vi "MasterAcquisitionFile_IOS_GCaMP_Garborg.vi"() -> ()   [LabVIEW 2020]
uses:
  <vilib>/vision/driver/IMAQdx.llb/IMAQdx Camera Control Mode.ctl
  <vilib>/vision/driver/IMAQdx.llb/IMAQdx Acquisition Mode.ctl
  <vilib>/userDefined/High Color/IMAQdx.ctl
  <vilib>/vision/driver/IMAQdx.llb/IMAQdx Buffer Number Mode.ctl
  <vilib>/DAQmx/write.llb/DAQmx Write (Digital 1D Wfm NChan NSamp).vi
  <vilib>/DAQmx/write.llb/DAQmx Write (Digital Bool 1Line 1Point).vi
  <vilib>/DAQmx/read.llb/DAQmx Read (Analog 1D Wfm NChan NSamp).vi
  <vilib>/Waveform/DWDTOps.llb/DWDT Digital to Boolean Array.vi
  <vilib>/DAQmx/create/channels.llb/DAQmx Create Channel (CO-Pulse Generation-Frequency).vi
  <vilib>/DAQmx/configure/timing.llb/DAQmx Timing (Implicit).vi
  <vilib>/DAQmx/create/channels.llb/DAQmx Create Channel (AI-Voltage-Basic).vi
  <vilib>/DAQmx/configure/timing.llb/DAQmx Timing (Sample Clock).vi
  <vilib>/DAQmx/configure/trigger.llb/DAQmx Start Trigger (Digital Edge).vi
  <vilib>/DAQmx/create/channels.llb/DAQmx Create Channel (DO-Digital Output).vi
  <vilib>/Waveform/DWDTOps.llb/DWDT Boolean Array to Digital.vi
  <vilib>/Waveform/DWDTOps.llb/DWDT Uncompress Digital.vi
  <vilib>/DAQmx/miscellaneous.llb/DAQmx Fill In Error Info.vi
  <vilib>/vision/driver/NI_Vision_Acquisition_Software.lvlib
  <resource>/objmgr/imaqdx.rc
  <resource>/objmgr/daqmx.rc
panel:
  out "LED":bool
  out "Auditory":bool
  out "RPad":bool
  out "LPad":bool
  out "Finished":bool
  in  "Generate Stimuli":bool
  in  "Sol Stim Parameters":cluster{"Fs":dbl, "Samples":dbl}
  in  "LED Stim Parameters":cluster{"Fs":dbl, "Samples":dbl}
  in  "Sol Duty Cycle (%)":dbl=50.0
  in  "Sol Freq":dbl=5.0
  in  "Sol Dur (s)":dbl=5.0
  in  "LED Duty Cycle (%)":dbl=10.0
  in  "LED Freq":dbl=10.0
  in  "LED Dur (s)":dbl=2.0
  out "Stimulus Order":digitalwaveform[](graph)=[{"t0"=timestamp(0 s since 1904-01-01), "dt"=5e-05, "Y"={"transitions"=[], "data"=array6001000x1[6001000 elements]}}, {"t0"=timestamp(0 s since 1904-01-01), "dt"=5e-05, "Y"={"transitions"=[], "data"=array6001000x1[6001000 elements]}}, {"t0"=timestamp(0 s since 1904-01-01), "dt"=5e-05, "Y"={"transitions"=[], "data"=array6001000x1[6001000 elements]}}, {"t0"=timestamp(0 s since 1904-01-01), "dt"=5e-05, "Y"={"transitions"=[], "data"=array6001000x1[6001000 elements]}}]
  out "Solenoid Stim":digitalwaveform(graph)={"t0"=timestamp(0 s since 1904-01-01), "dt"=5e-05, "Y"={"transitions"=[], "data"=array100000x1[100000 elements]}}
  in  "Trial Offset (s)":dbl=15.0
  in  "Interstim (s)":dbl=45.0
  in  "Right Pad":dbl=1.0
  in  "Left Pad":dbl=1.0
  in  "Auditory":dbl=1.0
  in  "LED":dbl
  out "?":T1(plugin-control)
  out "?":T1(plugin-control)
  out "?":T1(plugin-control)
  out "?":T1(plugin-control)
  in  "stop":bool
  out "CBV Cam":bool=TRUE
  out "Pupil Cam":bool=TRUE
  out "Whisk Cam":bool=TRUE
  out "Web Cam":bool=TRUE
  out "Analog":bool=TRUE
  out "Web Cam Fs":dbl(knob)=16.125821222377066 scale=0.0..200.0
  out "CBV Cam Fs":dbl(knob)=30.0 scale=0.0..200.0
  out "Whisk Cam Fs":dbl(knob)=150.0 scale=0.0..200.0
  out "Last Whisk\nBuffer 2":u32=891
  out "Pupil Cam Fs":dbl(knob)=30.0 scale=0.0..200.0
  out "Dropped 2":u32(slide) caption="Pupil Cam" scale=0.0..99.0
  out "Dev1 Samples":i32=594659
  in  "Dev1 Analog Channels":string[](array[string])=["Cortical_LH", "Force_Sensor", "LPadSol", "RPadSol", "AudSol", "Hippocampus", "EMG", "Cortical_RH", "OptoLED"]
  in  "Analog Acquisition":cluster{"Analog Fs":u16}={"Analog Fs"=20000} {"Analog Fs" format="%0.0f"}
  in  "Sampling Rates":T2={"Web Cam Fs"=30, "Whisk Cam Fs"=150, "Pupil Cam Fs"=30, "CBV Cam Fs"=30}
  out "Notes Size":i32=8
  out "Notes Reversed":string[](array[string])=["Experimenter", "Animal ID", "Hemisphere", "Solenoid PSI", "Isoflurane time", "Session ID", "Amplifier Gain", "LED power (mW)"]
  out "Notes Array":string[](array[string])=["LED power (mW)", "Amplifier Gain", "Session ID", "Isoflurane time", "Solenoid PSI", "Hemisphere", "Animal ID", "Experimenter"]
  in  "Notes:":T3={"Experimenter"="Kevin", "Animal ID"="T240", "Hemisphere"="Both", "Solenoid PSI"="10", "Isoflurane time"="1035", "Session ID"="Imaging Session One", "Amplifier Gain"="10000", "LED power (mW)"="10"}
  in  "Target Path":path=path "D:/T240" caption="Final Save Location"
  out "Dropped":u32(slide) caption="Whisk Cam" scale=0.0..999.0
  out "Filename":string="211203_12_05_39"
  out "CBV Camera":bool
  out "Time Elapsed (Min)":cluster{dbl, dbl}(slide)={5.0, 0.49561577000000007} scale=0.0..15.0 scale format="%#_2g"
  in  "Time (min)":dbl(knob)=5.0 min=0.5 max=20.0 step=0.5 scale=0.0..20.0 scale format="%#_2g"
  in  "Temp Path":path=path "D:/LabVIEW Streamed Data" caption="Temporary Path for Streamed Data"
  out "Last CBV\nBuffer":i32=891
  out "Last Whisk\nBuffer":u32=4458
  # "Dropped Frames"
  # "Stimuli"
  # "LPAD"
  # "RPAD"
  # "AUD"
  # "LED"
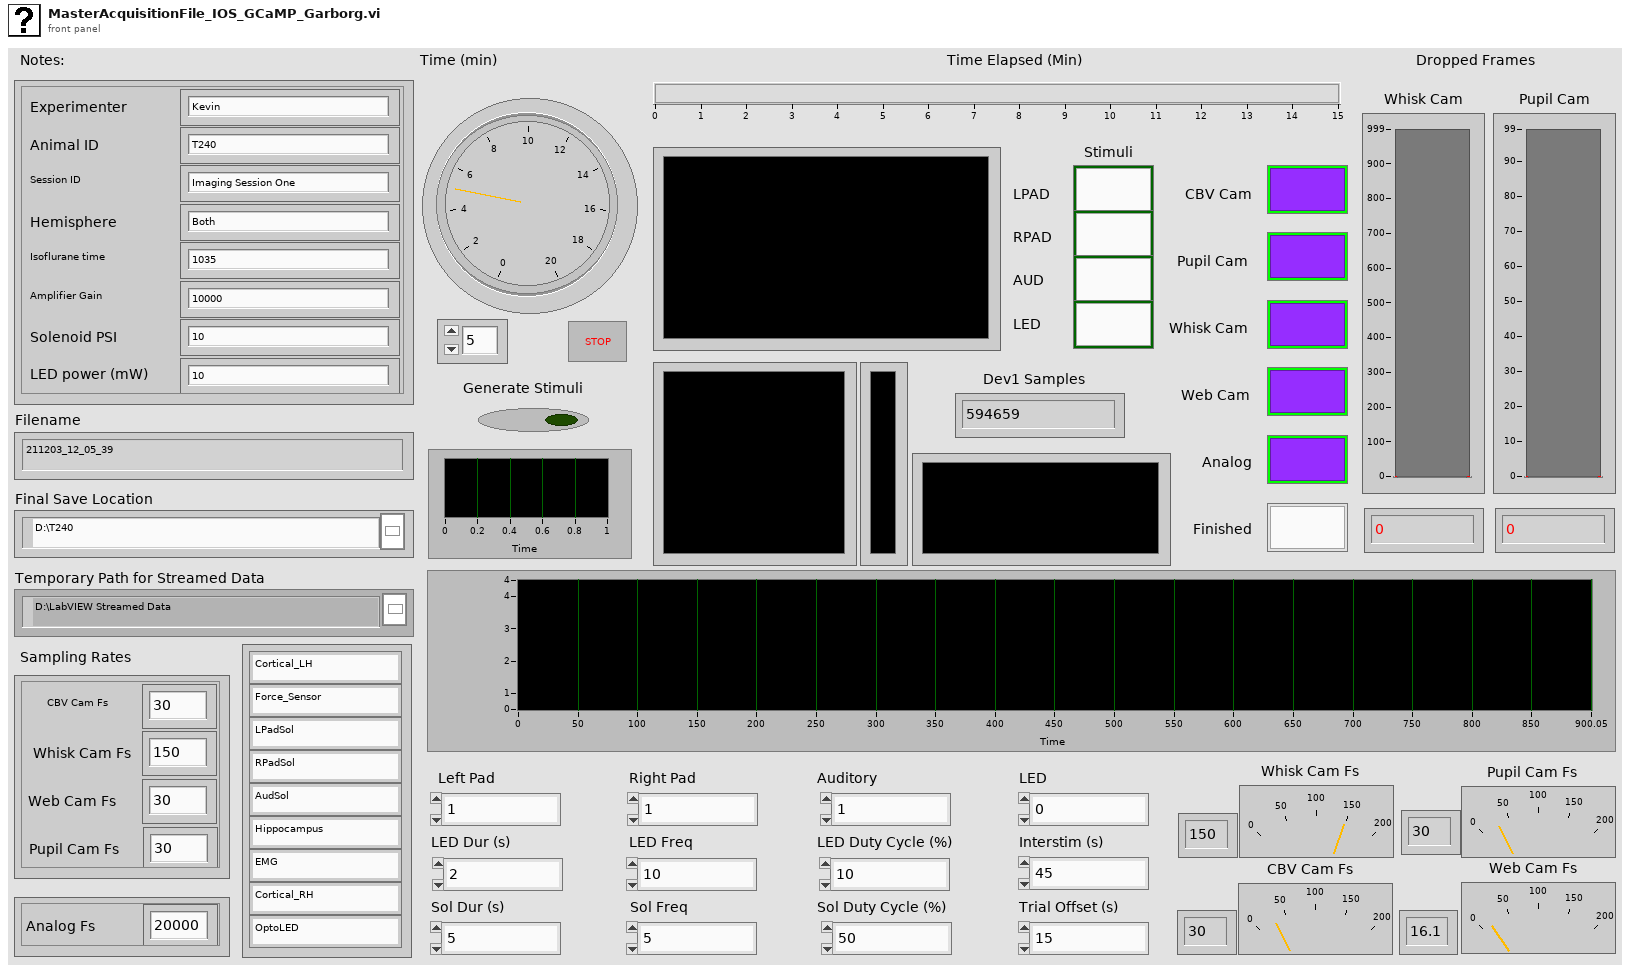
[diagram p1: front panel]
types:
  T1 = typedef "IMAQ Image.ctl" = refnum<image>
  T2 = cluster{"Web Cam Fs":u16, "Whisk Cam Fs":u16, "Pupil Cam Fs":u16, "CBV Cam Fs":u16}
  T3 = cluster{"Experimenter":string, "Animal ID":string, "Hemisphere":string, "Solenoid PSI":string, "Isoflurane time":string, "Session ID":string, "Amplifier Gain":string, "LED power (mW)":string}
  T4 = typedef "IMAQdx.ctl" = refnum<k21>
  T5 = enum16{"open", "replace", "create", "open or create", "replace or create", "replace or create with confirmation"}
  T6 = typedef "Image Type" = u32
  T7 = typedef "NI_Vision_Acquisition_Software.lvlib/IMAQdx Acquisition Mode.ctl" = enum32{"One Shot", "Continuous"}
  T8 = typedef "NI_Vision_Acquisition_Software.lvlib/IMAQdx Camera Control Mode.ctl" = enum32{"Controller", "Listener"}
  T9 = enum16{"open", "open or create", "create or replace", "create", "open (read-only)"}
  T10 = typedef "IMAQ AVI2 Refnum.ctl" = refnum<k20>
  T11 = enum16{"big-endian, network order", "native, host order", "little-endian"}
  T12 = typedef "NI_Vision_Acquisition_Software.lvlib/IMAQdx Buffer Number Mode.ctl" = enum32{"Next", "Last", "Buffer Number", "Every", "Last New"}
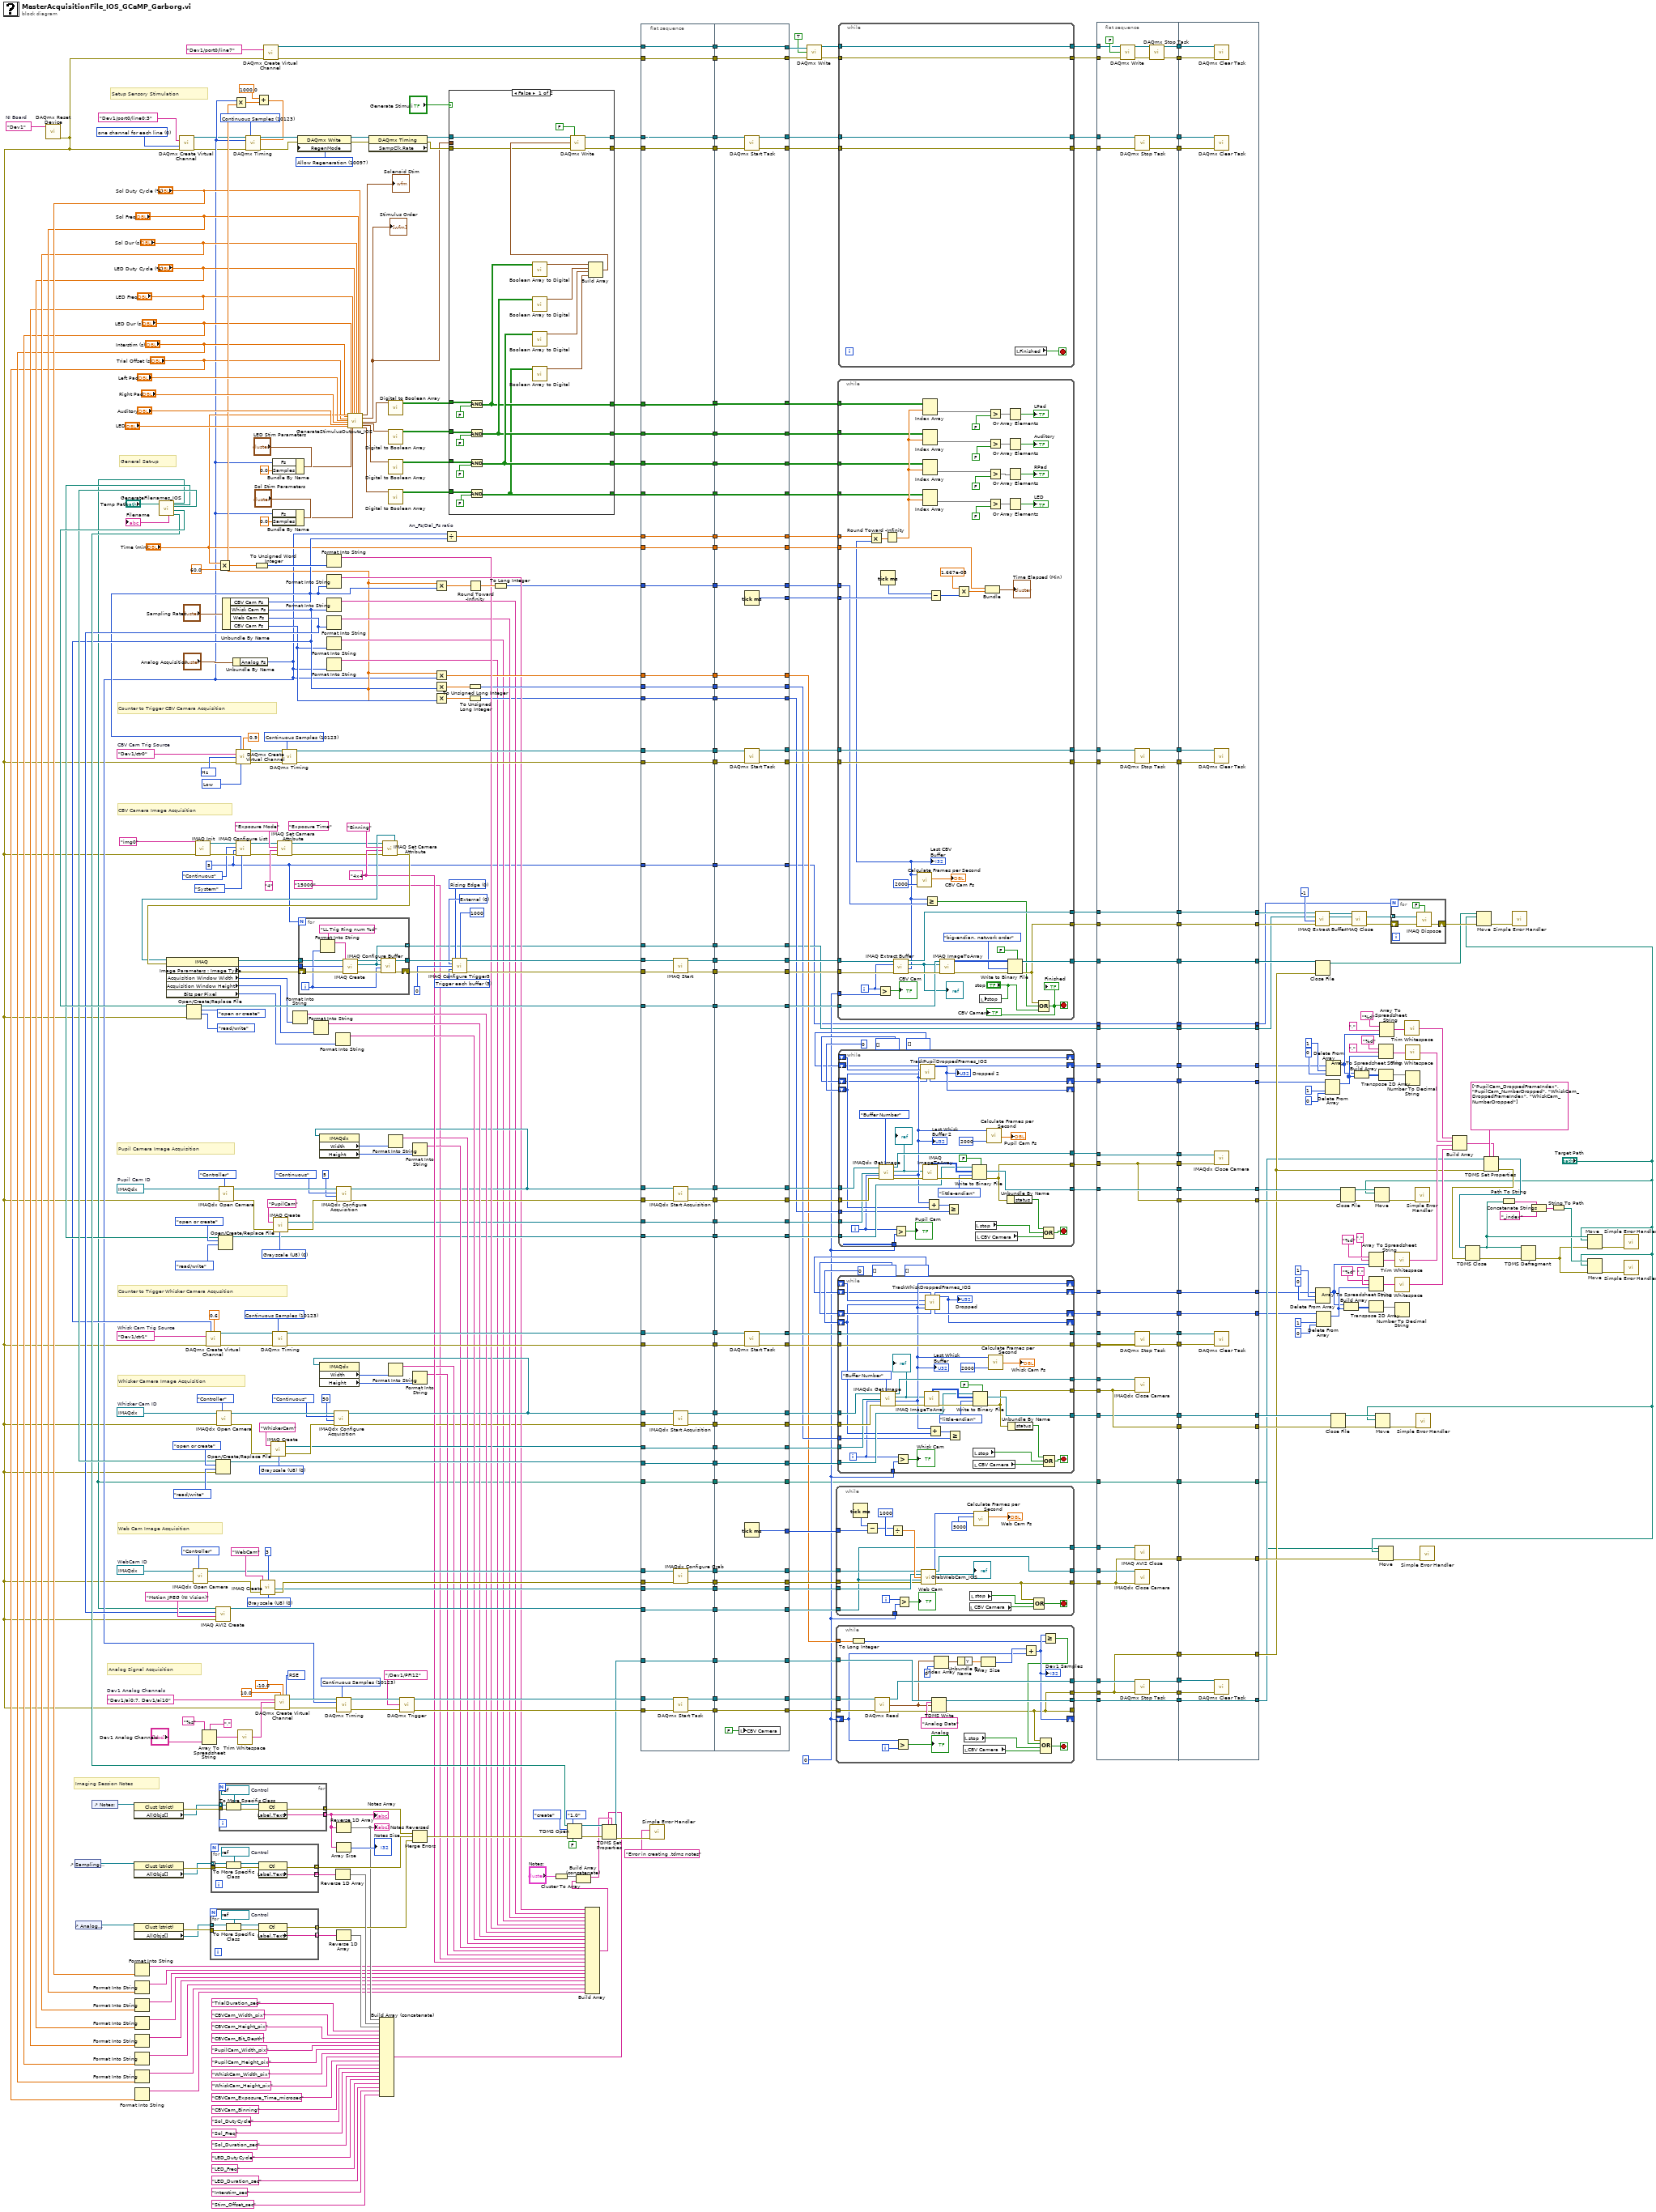
[diagram p0: block diagram]
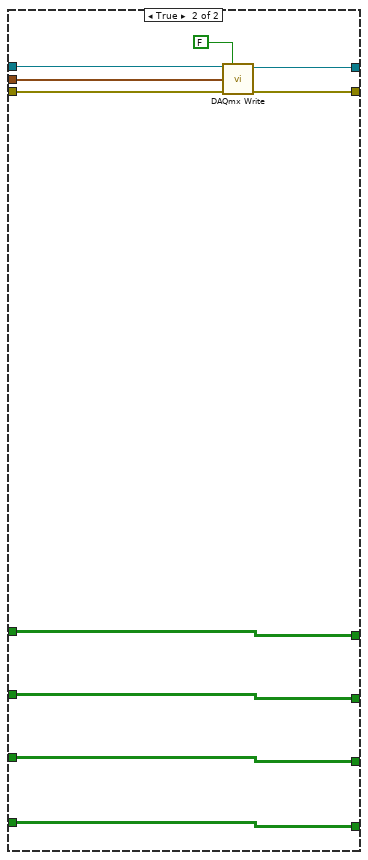
[diagram p2: hidden frame]
diagram:
  (unwired) "Exposure Time" ("Camera Attribute")
  w126 = 10097 items=["Allow Regeneration"=10097, "Do Not Allow Regeneration"=10158] ("RegenMode")
  w127 = 10123 items=["Finite Samples"=10178, "Continuous Samples"=10123, "Hardware Timed Single Point"=12522] ("sample mode")
  w130 = 0 items=["one channel for each line", "one channel for all lines"] ("line grouping")
  w324 = tag "Dev1/ai0:7, Dev1/ai10"  # Dev1 Analog Channels
  w327 = T4 "cam3"  # WebCam ID
  w305 = T4 "cam1"  # Whisker Cam ID
  w481 = tag "Dev1/ctr1"  # Whisk Cam Trig Source
  w255 = T4 "cam2"  # Pupil Cam ID
  w92 = tag "Dev1/ctr0"  # CBV Cam Trig Source
  w258 = T6 0 items=["Grayscale (U8)", "Grayscale (I16)", "Grayscale (SGL)", "Complex (CSG)", "RGB (U32)", "HSL (U32)", "RGB (U64)", "Grayscale (U16)"] ("Image Type")
  w245 = "4x4" ("Attribute Value")
  w183 = 0
  w400 = 10123 items=["Finite Samples"=10178, "Continuous Samples"=10123, "Hardware Timed Single Point"=12522] ("sample mode")
  w403 = 10083 items=["default"=-1, "RSE"=10083, "NRSE"=10078, "Differential"=10106, "Pseudodifferential"=12529] ("input terminal configuration")
  w447 = T6 0 items=["Grayscale (U8)", "Grayscale (I16)", "Grayscale (SGL)", "Complex (CSG)", "RGB (U32)", "HSL (U32)", "RGB (U64)", "Grayscale (U16)"] ("Image Type")
  w463 = u32 0 items=["Rising Edge", "Falling Edge"] ("Trigger Polarity")
  w466 = u32 0 items=["External"=0, "RTSI"=1, "ISO In"=2, "Scaled Encoder"=5] ("Trigger Type")
  w457 = tag "Dev1"  # NI Board
  w458 = 10123 items=["Finite Samples"=10178, "Continuous Samples"=10123, "Hardware Timed Single Point"=12522] ("sample mode")
  w461 = 10373 items=["Hz"=10373] ("units")
  w462 = 10214 items=["High"=10192, "Low"=10214] ("idle state")
  w25 = u32 5 ("Number of Buffers")
  w464 = u32 3 items=["Disabled", "Trigger start of acquisition", "Trigger start of each buffer list", "Trigger each buffer", "Trigger each line (linescan)", "Trigger end of acquisition"] ("Action")
  w477 = 10123 items=["Finite Samples"=10178, "Continuous Samples"=10123, "Hardware Timed Single Point"=12522] ("sample mode")
  w484 = T6 0 items=["Grayscale (U8)", "Grayscale (I16)", "Grayscale (SGL)", "Complex (CSG)", "RGB (U32)", "HSL (U32)", "RGB (U64)", "Grayscale (U16)"] ("Image Type")
  # "General Set-up"
  # "Pupil Camera Image Acquisition"
  # "Whisker Camera Image Acquisition"
  # "Imaging Session Notes"
  # "Setup Sensory Stimulation"
  # "CBV Camera Image Acquisition"
  # "Counter to Trigger CBV Camera Acquisition"
  # "Counter to Trigger Whisker Camera Acqusition"
  # "Web Cam Image Acquisition"
  # "Analog Signal Acquisition"
  n1 = call <vilib>:"DAQmx Reset Device.vi"("device in"=w457) -> ("error out"=w17:errorcluster)  [unwired: 14 in]
  n2 = control-ref of="Sampling Rates"() -> (w333:refnum<vi>)
  n3 = control-ref of="Analog Acquisition"() -> (w332:refnum<vi>)
  n4 = control-ref of="Notes:"() -> (w354:refnum<vi>)
  n5 = property class="Clust (strict)"(reference=w354) -> (error out=w357:errorcluster, "AllObjs[]"=w274:refnum<vi>[])  [unwired: 1 in, 1 out]
  n6 = property class="Clust (strict)"(reference=w333) -> (error out=w352:errorcluster, "AllObjs[]"=w275:refnum<vi>[])  [unwired: 1 in, 1 out]
  n7 = property class="Clust (strict)"(reference=w332) -> (error out=w331:errorcluster, "AllObjs[]"=w273:refnum<vi>[])  [unwired: 1 in, 1 out]
  n8 = Format Into String("Sol Duty Cycle (%)") -> (resulting string=w160:string)  [unwired: 3 in, 1 out]
  n9 = Format Into String("Sol Freq") -> (resulting string=w159:string)  [unwired: 3 in, 1 out]
  n10 = Format Into String("Sol Dur (s)") -> (resulting string=w158:string)  [unwired: 3 in, 1 out]
  n11 = Format Into String("LED Duty Cycle (%)") -> (resulting string=w157:string)  [unwired: 3 in, 1 out]
  n12 = Format Into String("LED Freq") -> (resulting string=w156:string)  [unwired: 3 in, 1 out]
  n13 = Format Into String("LED Dur (s)") -> (resulting string=w155:string)  [unwired: 3 in, 1 out]
  n14 = Format Into String("Interstim (s)") -> (resulting string=w154:string)  [unwired: 3 in, 1 out]
  n15 = Format Into String("Trial Offset (s)") -> (resulting string=w153:string)  [unwired: 3 in, 1 out]
  n16 = call "GenerateFilenames_IOS.vi"("path"="Temp Path") -> ("TDMS Path"=w349:path, "Dalsa Path"=w454:path, "Basler Path"=w450:path, "WebCam Path"=w19:path, "Analog file name"=→"Filename":string, "Basler2 Path"=w254:path)  [unwired: 3 in, 2 out]
  n17 = call-poly <vilib>:"DAQmx Create Virtual Channel.vi"("lines"=tag "Dev1/port0/line0:3", "line grouping"=w130, "error in"=w17) -> ("task out"=w129:refnum<k21>, "error out"=w128:errorcluster)  [unwired: 11 in]
  n18 = Open/Create/Replace File(file path (use dialog)=w454, error in=w17, operation (0:open)=T5."open or create", access (0:read/write)=enum16{"read/write", "read-only", "write-only"}."read/write") -> (refnum out=w404:refnum<file>)  [unwired: 2 in, 2 out]
  n19 = call <vilib>:"IMAQdx Open Camera.vi"("Camera Control Mode"=IMAQdx_Camera_Control_Mode."Controller", "error in"=w17, "Session In"=w327) -> ("error out"=w443:errorcluster, "Session Out"=w441:T4)  [unwired: 7 in]
  n20 = call <vilib>:"IMAQ Init.vi"("error in (no error)"=w17, "Interface Name"="img0") -> ("error out"=w475:errorcluster, "IMAQ Session Out"=w476:refnum<k11>)  [unwired: 8 out]
  n21 = Array To Spreadsheet String(delimiter (Tab)=",", array="Dev1 Analog Channels", 3:"%s" ("format string")) -> (spreadsheet string=w321:string)
  n22 = for {
    tunnel: [w496] -> w329 mode=indexing
    tunnel: w331 -> [w495]
    tunnel: [w493] -> w330 mode=indexing
    tunnel: w273 -> [w492] mode=indexing
    w497 = refnum<vi> refnum  # Control
    n23 = To More Specific Class(target class=w497, reference=w492, error in=w495) -> (specific class reference=w498:refnum<vi>, error out=w494:errorcluster)
    n24 = property class="Ctl"(reference=w498, error in=w494) -> (error out=w493:errorcluster, "Label.Text"=w496:string)  [unwired: 1 out]
  }
  n25 = for {
    tunnel: [w503] -> w353 mode=indexing
    tunnel: w352 -> [w502]
    tunnel: [w500] -> w339 mode=indexing
    tunnel: w275 -> [w499] mode=indexing
    w504 = refnum<vi> refnum  # Control
    n26 = To More Specific Class(target class=w504, reference=w499, error in=w502) -> (specific class reference=w505:refnum<vi>, error out=w501:errorcluster)
    n27 = property class="Ctl"(reference=w505, error in=w501) -> (error out=w500:errorcluster, "Label.Text"=w503:string)  [unwired: 1 out]
  }
  n28 = Open/Create/Replace File(file path (use dialog)=w450, error in=w17, operation (0:open)=T5."open or create", access (0:read/write)=enum16{"read/write", "read-only", "write-only"}."read/write") -> (refnum out=w420:refnum<file>)  [unwired: 2 in, 2 out]
  n29 = call <vilib>:"IMAQdx Open Camera.vi"("Camera Control Mode"=IMAQdx_Camera_Control_Mode."Controller", "error in"=w17, "Session In"=w305) -> ("error out"=w487:errorcluster, "Session Out"=w490:T4)  [unwired: 7 in]
  n30 = Multiply(x="Time (min)", y=60.0) -> (x*y=w170:dbl)
  n31 = Open/Create/Replace File(file path (use dialog)=w254, operation (0:open)=T5."open or create", access (0:read/write)=enum16{"read/write", "read-only", "write-only"}."read/write") -> (refnum out=w236:refnum<file>)  [unwired: 3 in, 2 out]
  n32 = call <vilib>:"IMAQdx Open Camera.vi"("Camera Control Mode"=IMAQdx_Camera_Control_Mode."Controller", "error in"=w17, "Session In"=w255) -> ("error out"=w261:errorcluster, "Session Out"=w264:T4)  [unwired: 7 in]
  n33 = for {
    tunnel: [w510] -> w356 mode=indexing
    tunnel: w357 -> [w509]
    tunnel: [w507] -> w340 mode=indexing
    tunnel: w274 -> [w506] mode=indexing
    w511 = refnum<vi> refnum  # Control
    n34 = To More Specific Class(target class=w511, reference=w506, error in=w509) -> (specific class reference=w512:refnum<vi>, error out=w508:errorcluster)
    n35 = property class="Ctl"(reference=w512, error in=w508) -> (error out=w507:errorcluster, "Label.Text"=w510:string)  [unwired: 1 out]
  }
  "Notes Array" <- w356
  n36 = Unbundle By Name("Sampling Rates") -> ("CBV Cam Fs"=w171:u16, "Whisk Cam Fs"=w225:u16, "Web Cam Fs"=w326:u16, "CBV Cam Fs"=w219:u16)
  n37 = call-poly <vilib>:"DAQmx Create Virtual Channel.vi"("frequency"=w225, "duty cycle"=0.6, "counter"=w481, "error in"=w17) -> ("task out"=w479:refnum<k21>, "error out"=w478:errorcluster)  [unwired: 10 in]
  n38 = call "IMAQ AVI2 Create"("error in (no error)"=w17, "Codec"="Motion JPEG (NI Vision)", "Frames Per Second"=w326, "AVI Path"=w19) -> ("AVI Refnum"=w433:T10)  [unwired: 6 in, 1 out]
  n39 = Unbundle By Name("Analog Acquisition") -> ("Analog Fs"=w143:u16)
  n40 = Multiply(x=w143, y=w170) -> (x*y=w103:dbl)
  n41 = call-poly <vilib>:"DAQmx Create Virtual Channel.vi"("frequency"=w171, "duty cycle"=0.9, "counter"=w92, "units"=w461, "error in"=w17, "idle state"=w462) -> ("task out"=w460:refnum<k21>, "error out"=w459:errorcluster)  [unwired: 8 in]
  n42 = call <vilib>:"IMAQ Configure List.vi"("Memory Location"=enum16{"System", "Onboard"}."System", "error in (no error)"=w475, "Number of buffers"=w25, "Continuous?"=enum16{"One-Shot", "Continuous"}."Continuous" ("Continuous ?"), "IMAQ Session In"=w476) -> ("error out"=w284:errorcluster, "IMAQ Session Out"=w282:refnum<k11>)  [unwired: 1 in, 4 out]
  n43 = call <vilib>:"Trim Whitespace.vi"("string"=w321) -> ("trimmed string"=w320:string)  [unwired: 1 in]
  n44 = To Unsigned Word Integer(number=w170) -> (unsigned 16bit integer=w316:u16)
  n45 = Add(x=1000.0, y=w103) -> (x+y=w101:dbl)
  n46 = call-poly <vilib>:"DAQmx Timing.vi"("task/channels in"=w129, "sample mode"=w127, "samples per channel"=w101, "rate"=w143, "error in"=w128) -> ("task out"=w123:refnum<k21>, "error out"=w122:errorcluster)  [unwired: 9 in]
  n47 = call "IMAQ Create"("Border Size"=3, "Image Name"="WebCam", "Image Type"=w447, "error in (no error)"=w443) -> ("New Image"=w440:T1, "error out"=w442:errorcluster)  [unwired: 1 in]
  n48 = call-poly <vilib>:"DAQmx Create Virtual Channel.vi"("lines"=tag "Dev1/port0/line7", "error in"=w17) -> ("task out"=w15:refnum<k21>, "error out"=w16:errorcluster)  [unwired: 12 in]
  n49 = call "IMAQ Create"("Image Name"="WhiskerCam", "Image Type"=w484, "error in (no error)"=w487) -> ("New Image"=w303:T1, "error out"=w485:errorcluster)  [unwired: 2 in]
  n50 = Bundle By Name(cluster="LED Stim Parameters", "Fs"=w143, "Samples"=0.0) -> (w176:cluster{"Fs":dbl, "Samples":dbl})
  n51 = Bundle By Name(cluster="Sol Stim Parameters", "Fs"=w143, "Samples"=0.0) -> (w177:cluster{"Fs":dbl, "Samples":dbl})
  n52 = call-poly <vilib>:"DAQmx Timing.vi"("task/channels in"=w479, "sample mode"=w477, "error in"=w478) -> ("task out"=w386:refnum<k21>, "error out"=w384:errorcluster)  [unwired: 11 in]
  n53 = call "IMAQ Create"("Image Name"="PupilCam", "Image Type"=w258, "error in (no error)"=w261) -> ("New Image"=w228:T1, "error out"=w259:errorcluster)  [unwired: 2 in]
  n54 = call-poly <vilib>:"DAQmx Create Virtual Channel.vi"("maximum value"=10.0, "minimum value"=-10.0, "input terminal configuration"=w403, "physical channels"=w324, "name to assign"=w320, "error in"=w17) -> ("task out"=w402:refnum<k21>, "error out"=w401:errorcluster)  [unwired: 8 in]
  n55 = call <vilib>:"IMAQ Set Camera Attribute.vi"("error in (no error)"=w284, "Attribute Value"="4", "Camera Attribute"="Exposure Mode", "IMAQ Session In"=w282) -> ("error out"=w1:errorcluster, "IMAQ Session Out"=w2:refnum<k11>)  [unwired: 4 in]
  n56 = call-poly <vilib>:"DAQmx Timing.vi"("task/channels in"=w460, "sample mode"=w458, "error in"=w459) -> ("task out"=w390:refnum<k21>, "error out"=w388:errorcluster)  [unwired: 11 in]
  n57 = property class="DAQmx Write"(reference=w123, error in=w122, "RegenMode"=w126) -> (reference out=w124:refnum<k21>, error out=w125:errorcluster)
  n58 = Format Into String(w316) -> (resulting string=w318:string)  [unwired: 3 in, 1 out]
  n59 = Format Into String(w171) -> (resulting string=w223:string)  [unwired: 3 in, 1 out]
  n60 = Format Into String(w225) -> (resulting string=w222:string)  [unwired: 3 in, 1 out]
  n61 = Format Into String(w326) -> (resulting string=w221:string)  [unwired: 3 in, 1 out]
  n62 = Format Into String(w219) -> (resulting string=w189:string)  [unwired: 3 in, 1 out]
  n63 = Format Into String(w143) -> (resulting string=w188:string)  [unwired: 3 in, 1 out]
  n64 = call <vilib>:"IMAQdx Configure Acquisition.vi"("error in"=w485, "Number of Buffers"=u32 50, "Continuous?"=IMAQdx_Acquisition_Mode."Continuous", "Session In"=w490) -> ("error out"=w196:errorcluster, "Session Out"=w304:T4)  [unwired: 6 in]
  n65 = property class="IMAQdx"(reference=w304) -> ("Width"=w315:u32, "Height"=w314:u32)  [unwired: 1 in, 2 out]
  n66 = Reverse 1D Array(array=w353) -> (reversed array=w343:string[])
  n67 = Reverse 1D Array(array=w356) -> (reversed array=w272:string[])
  "Notes Reversed" <- w272
  n68 = Array Size(array=w356) -> (size(s)=→"Notes Size":i32)
  n69 = Reverse 1D Array(array=w329) -> (reversed array=w328:string[])
  n70 = call <vilib>:"IMAQdx Configure Acquisition.vi"("error in"=w259, "Number of Buffers"=u32 5, "Continuous?"=IMAQdx_Acquisition_Mode."Continuous", "Session In"=w264) -> ("error out"=w238:errorcluster, "Session Out"=w229:T4)  [unwired: 6 in]
  n71 = property class="IMAQdx"(reference=w229) -> ("Width"=w253:u32, "Height"=w252:u32)  [unwired: 1 in, 2 out]
  n72 = call-poly <vilib>:"DAQmx Timing.vi"("task/channels in"=w402, "sample mode"=w400, "rate"=w143, "error in"=w401) -> ("task out"=w271:refnum<k21>, "error out"=w399:errorcluster)  [unwired: 10 in]
  n73 = call "GenerateStimulusOutputs_IOS.vi"("Trial duration (min)"="Time (min)", "Rest duration(s)"="Interstim (s)", "trial offset (s)"="Trial Offset (s)", "Left Pad"="Left Pad", "Right Pad"="Right Pad", "Auditory"="Auditory", "LED"="LED", "LED Stim Duration (s)"="LED Dur (s)", "LED Stim Parameters"=w176, "LED Frequency"="LED Freq", "Sol Stim Parameters"=w177, "LED duty cycle (%)"="LED Duty Cycle (%)", "Sol Stim Duration (s)"="Sol Dur (s)", "Sol Frequency"="Sol Freq", "Sol Duty Cycle (%)"="Sol Duty Cycle (%)") -> ("Solenoid Stim Waveforms"=→"Solenoid Stim":digitalwaveform, "Stimulus Digital Outputs"=w104:digitalwaveform[], "Left Pad Out"=w134:digitalwaveform, "Auditory Out"=w133:digitalwaveform, "Right Pad Out"=w132:digitalwaveform, "LED Out"=w131:digitalwaveform)  [unwired: 7 in]
  "Stimulus Order" <- w104
  n74 = property class="DAQmx Timing" props=["SampClk.Rate"](reference=w124, error in=w125) -> (reference out=w120:refnum<k21>, error out=w119:errorcluster)  [unwired: 1 out]
  n75 = Build Array (concatenate)(w272, w343, w328, "TrialDuration_sec", "CBVCam_Width_pix", "CBVCam_Height_pix", "CBVCam_Bit_Depth", "PupilCam_Width_pix", "PupilCam_Height_pix", "WhiskCam_Width_pix", "WhiskCam_Height_pix", "CBVCam_Exposure_Time_microsec" ("element"), "CBVCam_Binning" ("element"), "Sol_DutyCycle", "Sol_Freq", "Sol_Duration_sec", "LED_DutyCycle", "LED_Freq", "LED_Duration_sec", "Interstim_sec", "Stim_Offset_sec") -> (w266:string[])
  n76 = call <vilib>:"IMAQ Set Camera Attribute.vi"("error in (no error)"=w1, "Attribute Value"=w245, "Camera Attribute"="Binning", "IMAQ Session In"=w2) -> ("error out"=w283:errorcluster, "IMAQ Session Out"=w281:refnum<k11>)  [unwired: 4 in]
  n77 = property class="IMAQ"(reference=w281, error in=w283) -> (reference out=w290:refnum<k11>, error out=w289:errorcluster, "Image Parameters : Image Type"=w471:u32, "Acquisition Window Width"=w313:u32, "Acquisition Window Height"=w312:u32, "Bits per Pixel"=w311:u32)
  n78 = Format Into String(w313) -> (resulting string=w310:string)  [unwired: 3 in, 1 out]
  n79 = for {
    N: w25 -> [_]
    tunnel: [w522] -> w468
    tunnel: w471 -> [w520]
    shift-right: [w521] -> w467
    shift-left: w289 -> [w519]
    tunnel: [w514] -> w30 mode=indexing
    tunnel: w290 -> [w513]
    i -> [w515]
    n80 = Format Into String(format string="LL Trig Ring num %d", w515) -> (resulting string=w517:string)  [unwired: 2 in, 1 out]
    n81 = call "IMAQ Create"("Image Name"=w517, "Image Type"=w520, "error in (no error)"=w519) -> ("New Image"=w514:T1, "error out"=w518:errorcluster)  [unwired: 1 in, 1 out]
    n82 = call <vilib>:"IMAQ Configure Buffer.vi"("error in (no error)"=w518, "Buffer Number"=w515, "Image In"=w514, "IMAQ Session In"=w513) -> ("error out"=w521:errorcluster, "IMAQ Session Out"=w522:refnum<k11>)  [unwired: 2 in, 4 out]
  }
  n83 = Format Into String(w312) -> (resulting string=w268:string)  [unwired: 3 in, 1 out]
  n84 = Format Into String(w311) -> (resulting string=w309:string)  [unwired: 3 in, 1 out]
  n85 = Format Into String(w253) -> (resulting string=w241:string)  [unwired: 3 in, 1 out]
  n86 = Format Into String(w315) -> (resulting string=w243:string)  [unwired: 3 in, 1 out]
  n87 = call-poly <vilib>:"Digital to Boolean Array.vi"("digital waveform"=w134) -> ("boolean array"=w112:bool[][])  [unwired: 9 in, 1 out]
  n88 = call-poly <vilib>:"Digital to Boolean Array.vi"("digital waveform"=w133) -> ("boolean array"=w111:bool[][])  [unwired: 9 in, 1 out]
  n89 = call-poly <vilib>:"Digital to Boolean Array.vi"("digital waveform"=w132) -> ("boolean array"=w110:bool[][])  [unwired: 9 in, 1 out]
  n90 = call-poly <vilib>:"Digital to Boolean Array.vi"("digital waveform"=w131) -> ("boolean array"=w109:bool[][])  [unwired: 9 in, 1 out]
  n91 = call-poly <vilib>:"DAQmx Trigger.vi"("task/channels in"=w271, "source"=tag "/Dev1/PFI12", "error in"=w399) -> ("task out"=w398:refnum<k21>, "error out"=w397:errorcluster)  [unwired: 11 in]
  n92 = Format Into String(w252) -> (resulting string=w242:string)  [unwired: 3 in, 1 out]
  n93 = Format Into String(w314) -> (resulting string=w244:string)  [unwired: 3 in, 1 out]
  n94 = Merge Errors(w340, w339, w330) -> (w338:errorcluster)
  n95 = Multiply(x=w170, y=w171) -> (x*y=w452:dbl)
  n96 = Multiply(x=w170, y=w143) -> (x*y=w294:dbl)
  n97 = Multiply(x=w225, y=w170) -> (x*y=w269:dbl)
  n98 = Multiply(x=w219, y=w170) -> (x*y=w224:dbl)
  n99 = Divide "An_Fs/Dal_Fs ratio"(x=w143, y=w171) -> (x/y=w87:dbl)
  n100 = case shown="False" "Generate Stimuli" {
    tunnel: w120 -> [w533 w554]
    tunnel: w119 -> [w532 w553]
    tunnel: [w530 w552] -> w117
    tunnel: [w531 w551] -> w115
    tunnel: w112 -> [w541 w550]
    tunnel: w111 -> [w542 w549]
    tunnel: w110 -> [w543 w548]
    tunnel: w109 -> [w544 w547]
    tunnel: [w525 w550] -> w108
    tunnel: [w526 w549] -> w107
    tunnel: [w527 w548] -> w106
    tunnel: [w523 w547] -> w105
    tunnel: w104 -> [_ w546]
    frame False {
      n101 = Compound Arithmetic op=AND(w541, FALSE) -> (w525:bool[][])
      n102 = Compound Arithmetic op=AND(w542, FALSE) -> (w526:bool[][])
      n103 = Compound Arithmetic op=AND(w543, FALSE) -> (w527:bool[][])
      n104 = Compound Arithmetic op=AND(w544, FALSE) -> (w523:bool[][])
      n105 = call-poly <vilib>:"Boolean Array to Digital.vi"("boolean array"=w525) -> ("digital waveform"=w535:digitalwaveform)  [unwired: 9 in, 1 out]
      n106 = call-poly <vilib>:"Boolean Array to Digital.vi"("boolean array"=w526) -> ("digital waveform"=w529:digitalwaveform)  [unwired: 9 in, 1 out]
      n107 = call-poly <vilib>:"Boolean Array to Digital.vi"("boolean array"=w527) -> ("digital waveform"=w528:digitalwaveform)  [unwired: 9 in, 1 out]
      n108 = call-poly <vilib>:"Boolean Array to Digital.vi"("boolean array"=w523) -> ("digital waveform"=w524:digitalwaveform)  [unwired: 9 in, 1 out]
      n109 = Build Array(w535, w529, w528, w524) -> (w534:digitalwaveform[])
      n110 = call-poly <vilib>:"DAQmx Write.vi"("task/channels in"=w533, "auto start"=FALSE, "data"=w534, "error in"=w532) -> ("task out"=w530:refnum<k21>, "error out"=w531:errorcluster)  [unwired: 9 in, 1 out]
    }
    frame True {
      n111 = call-poly <vilib>:"DAQmx Write.vi"("task/channels in"=w554, "auto start"=FALSE, "data"=w546, "error in"=w553) -> ("task out"=w552:refnum<k21>, "error out"=w551:errorcluster)  [unwired: 9 in, 1 out]
    }
  }
  n112 = call <vilib>:"IMAQ Configure Trigger3.vi"("IMAQ Session In"=w468, "Polarity"=w463, "Frame timeout (ms)"=u32 1000 ("Frame Timeout (ms)"), "Type"=w466, "Line Number"=u32 0 ("Trigger Line Number"), "Action"=w464, "error in (no error)"=w467) -> ("IMAQ Session Out"=w419:refnum<k11>, "error out"=w418:errorcluster)  [unwired: 2 in, 5 out]
  n113 = To Unsigned Long Integer(number=w269) -> (unsigned 32bit integer=w292:u32)
  n114 = To Unsigned Long Integer(number=w224) -> (unsigned 32bit integer=w220:u32)
  n115 = Round Toward -Infinity(1:w452) -> (0:w451:dbl)
  n116 = To Long Integer(number=w451) -> (32bit integer=w197:i32)
  n117 = Cluster To Array(cluster="Notes:") -> (array=w350:string[])
  n118 = TDMS Open(6:FALSE ("disable buffering? (T)"), 7:enum16{"1.0", "2.0"}."1.0" ("file format version (2.0)"), 8:w338, 10:T9."create" ("operation (0:open)"), 11:w349) -> (0:w344:errorcluster, 3:w345:refnum<k34>)  [unwired: 2 in]
  n119 = Build Array(w223, w222, w221, w189, w188, w318, w310, w268, w309, w241, w242, w243, w244, "15000" ("Exposure Time (microsec)"), w245, w160, w159, w158, w157, w156, w155, w154, w153) -> (w325:string[])
  n120 = Build Array (concatenate)(w350, w325) -> (w342:string[])
  n121 = TDMS Set Properties(5:w342, 7:w266, 8:w344, 11:w345) -> (0:w337:errorcluster, 3:w341:refnum<k34>)  [unwired: 2 in, 2 out]
  n122 = flat-sequence {
    tunnel: w442 -> [w603]
    tunnel: w441 -> [w602]
    tunnel: w440 -> [w601]
    tunnel: [w601] -> w439
    tunnel: [w600] -> w437
    tunnel: [w599] -> w435
    tunnel: w433 -> [w598]
    tunnel: [w598] -> w432
    tunnel: w304 -> [w597]
    tunnel: w196 -> [w596]
    tunnel: [w595] -> w427
    tunnel: [w594] -> w425
    tunnel: [w593] -> w423
    tunnel: w303 -> [w593]
    tunnel: [w592] -> w421
    tunnel: w420 -> [w592]
    tunnel: w419 -> [w591]
    tunnel: w418 -> [w590]
    tunnel: [w589] -> w416
    tunnel: [w588] -> w414
    tunnel: w197 -> [w587]
    tunnel: [w587] -> w410
    tunnel: "Time (min)" -> [w586]
    tunnel: [w586] -> w407
    tunnel: [w585] -> w405
    tunnel: w404 -> [w585]
    tunnel: w398 -> [w584]
    tunnel: w397 -> [w583]
    tunnel: [w582] -> w396
    tunnel: [w581] -> w395
    tunnel: [w580] -> w391
    tunnel: w341 -> [w580]
    tunnel: w390 -> [w579]
    tunnel: [w579] -> w389
    tunnel: w388 -> [w578]
    tunnel: [w578] -> w387
    tunnel: w386 -> [w577]
    tunnel: [w577] -> w385
    tunnel: w384 -> [w576]
    tunnel: [w576] -> w383
    tunnel: w294 -> [w575]
    tunnel: [w575] -> w293
    tunnel: w292 -> [w574]
    tunnel: [w574] -> w291
    tunnel: [w569] -> w240
    tunnel: w229 -> [w570]
    tunnel: [w567] -> w239
    tunnel: w238 -> [w568]
    tunnel: [w573] -> w237
    tunnel: w236 -> [w573]
    tunnel: w228 -> [w572]
    tunnel: [w572] -> w227
    tunnel: w220 -> [w571]
    tunnel: [w571] -> w218
    tunnel: [w566] -> w142
    tunnel: w108 -> [w566]
    tunnel: [w565] -> w141
    tunnel: w107 -> [w565]
    tunnel: [w564] -> w140
    tunnel: w106 -> [w564]
    tunnel: [w563] -> w139
    tunnel: w105 -> [w563]
    tunnel: [w562] -> w118
    tunnel: w117 -> [w562]
    tunnel: [w561] -> w116
    tunnel: w115 -> [w561]
    tunnel: w87 -> [w560]
    tunnel: [w560] -> w86
    tunnel: w30 -> [w559]
    tunnel: [w559] -> w33
    tunnel: w25 -> [w558]
    tunnel: [w558] -> w28
    tunnel: w19 -> [w557]
    tunnel: [w557] -> w20
    tunnel: w16 -> [w555]
    tunnel: w15 -> [w556]
    tunnel: [w556] -> w13
    tunnel: [w555] -> w11
    tunnel: [w651] -> w444
    tunnel: w439 -> [w650]
    tunnel: [w650] -> w438
    tunnel: w437 -> [w649]
    tunnel: [w649] -> w436
    tunnel: w435 -> [w648]
    tunnel: [w648] -> w434
    tunnel: w432 -> [w647]
    tunnel: [w647] -> w431
    tunnel: [w629] -> w430
    tunnel: [w628] -> w429
    tunnel: [w646] -> w428
    tunnel: w427 -> [w646]
    tunnel: [w645] -> w426
    tunnel: w425 -> [w645]
    tunnel: [w644] -> w424
    tunnel: w423 -> [w644]
    tunnel: [w643] -> w422
    tunnel: w421 -> [w643]
    tunnel: [w642] -> w417
    tunnel: w416 -> [w642]
    tunnel: [w641] -> w415
    tunnel: w414 -> [w641]
    tunnel: [w633] -> w413
    tunnel: [w632] -> w412
    tunnel: [w640] -> w411
    tunnel: w410 -> [w639]
    tunnel: [w639] -> w409
    tunnel: [w638] -> w408
    tunnel: w407 -> [w638]
    tunnel: [w637] -> w406
    tunnel: w405 -> [w637]
    tunnel: [w636] -> w393
    tunnel: w396 -> [w636]
    tunnel: [w635] -> w394
    tunnel: w395 -> [w635]
    tunnel: [w634] -> w186
    tunnel: w391 -> [w634]
    tunnel: w389 -> [w631]
    tunnel: w387 -> [w630]
    tunnel: w385 -> [w627]
    tunnel: w383 -> [w626]
    tunnel: w293 -> [w625]
    tunnel: [w625] -> w187
    tunnel: w291 -> [w624]
    tunnel: [w624] -> w217
    tunnel: w240 -> [w622]
    tunnel: w239 -> [w621]
    tunnel: w237 -> [w620]
    tunnel: [w622] -> w232
    tunnel: [w621] -> w231
    tunnel: [w620] -> w230
    tunnel: [w619] -> w226
    tunnel: w227 -> [w619]
    tunnel: [w618] -> w216
    tunnel: w218 -> [w618]
    tunnel: w142 -> [w614]
    tunnel: w141 -> [w617]
    tunnel: w140 -> [w616]
    tunnel: w139 -> [w615]
    tunnel: [w614] -> w138
    tunnel: [w617] -> w137
    tunnel: [w616] -> w136
    tunnel: [w615] -> w135
    tunnel: w118 -> [w613]
    tunnel: w116 -> [w612]
    tunnel: [w611] -> w114
    tunnel: [w610] -> w113
    tunnel: w86 -> [w609]
    tunnel: [w609] -> w85
    tunnel: w33 -> [w608]
    tunnel: [w608] -> w32
    tunnel: w28 -> [w607]
    tunnel: [w607] -> w27
    tunnel: [w606] -> w22
    tunnel: w20 -> [w606]
    tunnel: [w605] -> w14
    tunnel: w13 -> [w605]
    tunnel: [w604] -> w12
    tunnel: w11 -> [w604]
    frame #0 {
      n123 = call <vilib>:"IMAQ Start.vi"("error in (no error)"=w590, "IMAQ Session In"=w591) -> ("error out"=w588:errorcluster, "IMAQ Session Out"=w589:refnum<k11>)  [unwired: 8 out]
      n124 = call <vilib>:"IMAQdx Start Acquisition.vi"("error in"=w568, "Session In"=w570) -> ("error out"=w567:errorcluster, "Session Out"=w569:T4)  [unwired: 8 in]
      n125 = call <vilib>:"IMAQdx Start Acquisition.vi"("error in"=w596, "Session In"=w597) -> ("error out"=w594:errorcluster, "Session Out"=w595:T4)  [unwired: 8 in]
      n126 = call <vilib>:"IMAQdx Configure Grab.vi"("error in"=w603, "Session In"=w602) -> ("error out"=w599:errorcluster, "Session Out"=w600:T4)  [unwired: 8 in]
      n127 = call <vilib>:"DAQmx Start Task.vi"("task/channels in"=w584, "error in"=w583) -> ("task out"=w582:refnum<k21>, "error out"=w581:errorcluster)  [unwired: 12 in]
    }
    frame #1 {
      n128 = local write "CBV Camera"(FALSE ("Finished Acquiring")) -> ()
      n129 = call <vilib>:"DAQmx Start Task.vi"("task/channels in"=w613, "error in"=w612) -> ("task out"=w611:refnum<k21>, "error out"=w610:errorcluster)  [unwired: 12 in]
      n130 = Tick Count (ms)() -> (millisecond timer value=w640:u32)
      n131 = call <vilib>:"DAQmx Start Task.vi"("task/channels in"=w631, "error in"=w630) -> ("task out"=w633:refnum<k21>, "error out"=w632:errorcluster)  [unwired: 12 in]
      n132 = call <vilib>:"DAQmx Start Task.vi"("task/channels in"=w627, "error in"=w626) -> ("task out"=w629:refnum<k21>, "error out"=w628:errorcluster)  [unwired: 12 in]
      n133 = Tick Count (ms)() -> (millisecond timer value=w651:u32)
    }
  }
  n134 = call <vilib>:"Simple Error Handler.vi"("error source (\" \")"="Error in creating .tdms notes" ("error source (\" \")"), "error in (no error)"=w337) -> ()  [unwired: 3 in, 5 out]
  n135 = call-poly <vilib>:"DAQmx Write.vi"("task/channels in"=w14, "data"=TRUE, "error in"=w12) -> ("task out"=w6:refnum<k21>, "error out"=w5:errorcluster)  [unwired: 10 in, 1 out]
  n136 = while {
    tunnel: w394 -> [w674]
    tunnel: w393 -> [w673]
    tunnel: w186 -> [w672]
    tunnel: [w671] -> w53
    tunnel: [w660] -> _
    tunnel: [w670] -> w84
    shift-right: [w664] -> _
    shift-left: w183 -> [w655]
    tunnel: [w660] -> w83
    tunnel: w187 -> [w658]
    i -> [w656]
    stop <- w661 stop-if-true
    n137 = To Long Integer(number=w658) -> (32bit integer=w659:i32)
    n138 = call-poly <vilib>:"DAQmx Read.vi"("task/channels in"=w673, "error in"=w674) -> ("task out"=w670:refnum<k21>, "data"=w652:waveform(dbl)[], "error out"=w663:errorcluster)  [unwired: 11 in]
    n139 = Greater?(x=w655, y=w656) -> (0:→"Analog":bool)
    n140 = TDMS Write(0:w672, 5:"Analog Data" ("group name in (Untitled)"), 9:w652, 11:w663) -> (4:w671:refnum<k34>, 15:w660:errorcluster)  [unwired: 2 in, 2 out]
    n141 = Index Array(array=w652, index=0) -> (element=w667:waveform(dbl))
    n142 = Unbundle By Name(w667) -> ("Y"=w666:dbl[])
    n143 = local read "CBV Camera"() -> (w654:bool)
    n144 = local read "stop"() -> (w653:bool)
    n145 = Array Size(array=w666) -> (size(s)=w665:i32)
    n146 = Add(x=w665, y=w655) -> (x+y=w664:i32)
    "Dev1 Samples" <- w664
    n147 = Greater Or Equal?(x=w664, y=w659) -> (x >= y?=w662:bool)
    n148 = Compound Arithmetic op=OR(w660, w662, w653, w654) -> (w661:bool)
  }
  n149 = while {
    tunnel: w444 -> [w691]
    tunnel: w438 -> [w689]
    tunnel: w436 -> [w688]
    tunnel: w434 -> [w687]
    tunnel: w431 -> [w685]
    tunnel: [w686] -> w75
    tunnel: [w677] -> w76
    tunnel: [w685] -> w74
    tunnel: w183 -> [w680]
    i -> [w681]
    stop <- w678 stop-if-true
    n150 = Tick Count (ms)() -> (millisecond timer value=w693:u32)
    n151 = Subtract(x=w693, y=w691) -> (x-y=w694:u32)
    n152 = Divide(x=w694, y=u32 1000) -> (x/y=w690:dbl)
    n153 = Greater?(x=w681, y=w680) -> (0:→"Web Cam":bool)
    n154 = call "GrabWebCam_IOS.vi"("Session In"=w688, "Image In"=w689, "Trial Time"=w690, "AVI Refnum"=w685, "error in"=w687) -> ("Session Out"=w686:T4, "WebCam Img Out"=→"?":T1, "Buffer Number Out"=w684:u32, "error out"=w677:errorcluster)  [unwired: 7 in]
    n155 = local read "CBV Camera"() -> (w679:bool)
    n156 = local read "stop"() -> (w676:bool)
    n157 = call <vilib>:"Calculate Frames per Second.vi"("Update Interval (ms)"=u32 5000, "Buffer Number"=w684) -> ("Processed Frames/s"=→"Web Cam Fs":dbl)  [unwired: 7 in, 2 out]
    n158 = Compound Arithmetic op=OR(w677, w676, w679) -> (w678:bool)
  }
  n159 = while {
    tunnel: w417 -> [w748]
    tunnel: w415 -> [w749]
    tunnel: [w731] -> w36
    tunnel: [w729] -> w39
    tunnel: [w743] -> w64
    tunnel: [w738] -> w96
    tunnel: w413 -> [w738]
    tunnel: [w737] -> w95
    tunnel: w412 -> [w737]
    tunnel: w411 -> [w736]
    tunnel: w409 -> [w735]
    tunnel: w408 -> [w734]
    tunnel: w406 -> [w728]
    tunnel: w183 -> [w723]
    tunnel: w138 -> [w707]
    tunnel: w137 -> [w708]
    tunnel: w136 -> [w702]
    tunnel: w135 -> [w699]
    tunnel: w85 -> [w696]
    i -> [w724]
    stop <- w718 stop-if-true
    n160 = Greater?(x=w724, y=w723) -> (0:→"CBV Cam":bool)
    n161 = Tick Count (ms)() -> (millisecond timer value=w741:u32)
    n162 = call <vilib>:"IMAQ Extract Buffer.vi"("error in (no error)"=w749, "Buffer to extract"=w724, "IMAQ Session In"=w748) -> ("error out"=w742:errorcluster, "Buffer Number"=w719:i32, "Image Out"=w721:T1, "IMAQ Session Out"=w729:refnum<k11>)  [unwired: 5 out]
    "Last CBV\nBuffer" <- w719
    "?" <- w721
    n163 = Multiply(x=w696, y=w719) -> (x*y=w720:dbl)
    n164 = Round Toward -Infinity(1:w720) -> (0:w713:dbl)
    n165 = call <vilib>:"Calculate Frames per Second.vi"("Update Interval (ms)"=u32 2000, "Buffer Number"=w719) -> ("Processed Frames/s"=→"CBV Cam Fs":dbl)  [unwired: 7 in, 2 out]
    n166 = Index Array(array=w707, index (row)=w713) -> (element=w706:bool[])  [unwired: 1 in]
    n167 = Index Array(array=w708, index (row)=w713) -> (element=w704:bool[])  [unwired: 1 in]
    n168 = Index Array(array=w702, index (row)=w713) -> (element=w701:bool[])  [unwired: 1 in]
    n169 = Index Array(array=w699, index (row)=w713) -> (element=w698:bool[])  [unwired: 1 in]
    n170 = Greater Or Equal?(x=w719, y=w735) -> (x >= y?=w727:bool)
    n171 = Subtract(x=w741, y=w736) -> (x-y=w740:u32)
    n172 = call "IMAQ ImageToArray"("error in (no error)"=w742, "Image"=w721) -> ("error out"=w747:errorcluster, "Image Pixels (I16)"=w746:i16[][])  [unwired: 2 in, 3 out]
    n173 = Multiply(x=w740, y=1.667e-05) -> (x*y=w739:dbl)
    n174 = local write "stop"("stop") -> ()
    n175 = Bundle("Time (min)"=w734, w739) -> (→"Time Elapsed (Min)":cluster{"Time (min)":dbl, dbl})  [unwired: 1 in]
    n176 = Greater?(x=w706, y=FALSE ("Boolean")) -> (0:w705:bool[])
    n177 = Greater?(x=w704, y=FALSE ("Boolean")) -> (0:w703:bool[])
    n178 = Greater?(x=w701, y=FALSE ("Boolean")) -> (0:w700:bool[])
    n179 = Greater?(x=w698, y=FALSE ("Boolean")) -> (0:w697:bool[])
    n180 = Or Array Elements(Boolean array=w705) -> (logical OR=→"LPad":bool)
    n181 = Or Array Elements(Boolean array=w703) -> (logical OR=→"Auditory":bool)
    n182 = Or Array Elements(Boolean array=w700) -> (logical OR=→"RPad":bool)
    n183 = Or Array Elements(Boolean array=w697) -> (logical OR=→"LED":bool)
    n184 = Write to Binary File(file (use dialog)=w728, data=w746, error in=w747, 5:FALSE ("prepend array or string size? (T)"), 9:T11."big-endian, network order" ("byte order (0:big-endian, network order)")) -> (refnum out=w743:refnum<file>, error out=w731:errorcluster)  [unwired: 1 in, 1 out]
    n185 = Compound Arithmetic op=OR(w731, w727, "stop") -> (w718:bool)
    "CBV Camera" <- w718
    "Finished" <- w718
  }
  n186 = while {
    tunnel: w430 -> [w776]
    tunnel: [w777] -> w79
    tunnel: w429 -> [w777]
    tunnel: [w776] -> w80
    tunnel: [w769] -> w70
    tunnel: [w770] -> w71
    tunnel: [w775] -> w66
    tunnel: w428 -> [w774]
    tunnel: w426 -> [w773]
    tunnel: w424 -> [w772]
    tunnel: w422 -> [w771]
    shift-right: [w760] -> _
    shift-left: _ -> [w758]
    shift-right: [w755] -> _
    shift-left: u32 0 ("New Lost") -> [w759]
    shift-right: [w756] -> w48
    shift-left: u32[] [] ("NewBuffNum") -> [w757]
    shift-right: [w762] -> w51
    shift-left: u32[] [] ("NewNumLost") -> [w761]
    tunnel: w217 -> [w767]
    tunnel: w183 -> [w763]
    i -> [w750]
    stop <- w766 stop-if-true
    n187 = call <vilib>:"IMAQdx Get Image.vi"("Buffer Number Mode (Next)"=IMAQdx_Buffer_Number_Mode."Buffer Number", "error in"=w773, "Buffer Number In"=w750, "Image In"=w772, "Session In"=w774) -> ("error out"=w783:errorcluster, "Buffer Number Out"=w760:u32, "Image Out"=w752:T1, "Session Out"=w769:T4)  [unwired: 3 in]
    "Last Whisk\nBuffer" <- w760
    "?" <- w752
    n188 = Greater?(x=w750, y=w763) -> (0:→"Whisk Cam":bool)
    n189 = call "IMAQ ImageToArray"("error in (no error)"=w783, "Image"=w752) -> ("error out"=w782:errorcluster, "Image Pixels (U8)"=w781:u8[][])  [unwired: 2 in, 3 out]
    n190 = call "TrackWhiskDroppedFrames_IOS.vi"("NumLost"=w761, "BuffNum"=w757, "Curr Buffer"=w760, "Prev Lost"=w759, "Prev Buffer"=w758) -> ("New Lost"=w755:u32, "NewNumLost"=w762:u32[], "NewBuffNum"=w756:u32[])  [unwired: 4 in]
    "Dropped" <- w755
    n191 = Add(x=w760, y=w759) -> (x+y=w768:u32)
    n192 = Greater Or Equal?(x=w768, y=w767) -> ()  [unwired: 1 out]
    n193 = Write to Binary File(file (use dialog)=w771, data=w781, error in=w782, 5:FALSE ("prepend array or string size? (T)"), 9:T11."little-endian" ("byte order (0:big-endian, network order)")) -> (refnum out=w775:refnum<file>, error out=w770:errorcluster)  [unwired: 1 in, 1 out]
    n194 = local read "stop"() -> (w754:bool)
    n195 = local read "CBV Camera"() -> (w753:bool)
    n196 = call <vilib>:"Calculate Frames per Second.vi"("Update Interval (ms)"=u32 2000, "Buffer Number"=w760) -> ("Processed Frames/s"=→"Whisk Cam Fs":dbl)  [unwired: 7 in, 2 out]
    n197 = Unbundle By Name(w770) -> ("status"=w751:bool)
    n198 = Compound Arithmetic op=OR(w751, w754, w753) -> (w766:bool)
  }
  n199 = while {
    tunnel: w114 -> [w787]
    tunnel: [w788] -> w99
    tunnel: w113 -> [w788]
    tunnel: [w787] -> w100
    tunnel: [w786] -> w7
    tunnel: w6 -> [w786]
    tunnel: w5 -> [w785]
    tunnel: [w785] -> w4
    stop <- w789 stop-if-true
    n200 = local read "Finished"() -> (w789:bool)
  }
  n201 = while {
    tunnel: [w804] -> w90
    tunnel: [w805] -> w89
    tunnel: [w814] -> w61
    tunnel: w232 -> [w813]
    tunnel: w231 -> [w812]
    tunnel: w226 -> [w811]
    tunnel: w230 -> [w810]
    shift-right: [w803] -> _
    shift-left: _ -> [w809]
    shift-right: [w808] -> _
    shift-left: u32 0 ("New Lost") -> [w802]
    shift-right: [w807] -> w42
    shift-left: u32[] [] ("NewBuffNum") -> [w798]
    shift-right: [w806] -> w45
    shift-left: u32[] [] ("NewNumLost") -> [w799]
    tunnel: w216 -> [w797]
    tunnel: w183 -> [w795]
    i -> [w790]
    stop <- w800 stop-if-true
    n202 = call <vilib>:"IMAQdx Get Image.vi"("Buffer Number Mode (Next)"=IMAQdx_Buffer_Number_Mode."Buffer Number", "error in"=w812, "Buffer Number In"=w790, "Image In"=w811, "Session In"=w813) -> ("error out"=w821:errorcluster, "Buffer Number Out"=w803:u32, "Image Out"=w792:T1, "Session Out"=w804:T4)  [unwired: 3 in]
    "Last Whisk\nBuffer 2" <- w803
    "?" <- w792
    n203 = Greater?(x=w790, y=w795) -> (0:→"Pupil Cam":bool)
    n204 = call "TrackPupilDroppedFrames_IOS.vi"("NumLost"=w799, "BuffNum"=w798, "Curr Buffer"=w803, "Prev Lost"=w802, "Prev Buffer"=w809) -> ("New Lost"=w808:u32, "NewNumLost"=w806:u32[], "NewBuffNum"=w807:u32[])  [unwired: 4 in]
    "Dropped 2" <- w808
    n205 = call "IMAQ ImageToArray"("error in (no error)"=w821, "Image"=w792) -> ("error out"=w820:errorcluster, "Image Pixels (U8)"=w819:u8[][])  [unwired: 2 in, 3 out]
    n206 = Add(x=w803, y=w802) -> (x+y=w801:u32)
    n207 = Greater Or Equal?(x=w801, y=w797) -> ()  [unwired: 1 out]
    n208 = Write to Binary File(file (use dialog)=w810, data=w819, error in=w820, 5:FALSE ("prepend array or string size? (T)"), 9:T11."little-endian" ("byte order (0:big-endian, network order)")) -> (refnum out=w814:refnum<file>, error out=w805:errorcluster)  [unwired: 1 in, 1 out]
    n209 = local read "stop"() -> (w794:bool)
    n210 = local read "CBV Camera"() -> (w793:bool)
    n211 = call <vilib>:"Calculate Frames per Second.vi"("Update Interval (ms)"=u32 2000, "Buffer Number"=w803) -> ("Processed Frames/s"=→"Pupil Cam Fs":dbl)  [unwired: 7 in, 2 out]
    n212 = Unbundle By Name(w805) -> ("status"=w791:bool)
    n213 = Compound Arithmetic op=OR(w791, w794, w793) -> (w800:bool)
  }
  n214 = flat-sequence {
    tunnel: w100 -> [w866]
    tunnel: w99 -> [w865]
    tunnel: [w864] -> w98
    tunnel: [w863] -> w97
    tunnel: w96 -> [w862]
    tunnel: w95 -> [w861]
    tunnel: [w860] -> w94
    tunnel: [w859] -> w93
    tunnel: [w858] -> w91
    tunnel: w90 -> [w858]
    tunnel: w89 -> [w841]
    tunnel: [w841] -> w88
    tunnel: w84 -> [w857]
    tunnel: w83 -> [w840]
    tunnel: [w856] -> w82
    tunnel: [w855] -> w81
    tunnel: w80 -> [w854]
    tunnel: w79 -> [w853]
    tunnel: [w852] -> _
    tunnel: [w851] -> _
    tunnel: [w852] -> w78
    tunnel: [w851] -> w77
    tunnel: w76 -> [w849]
    tunnel: w75 -> [w850]
    tunnel: w74 -> [w848]
    tunnel: [w847] -> w73
    tunnel: w71 -> [w845]
    tunnel: w70 -> [w846]
    tunnel: [w845] -> w68
    tunnel: [w844] -> w67
    tunnel: w66 -> [w844]
    tunnel: w64 -> [w843]
    tunnel: [w843] -> w63
    tunnel: w61 -> [w842]
    tunnel: [w842] -> w60
    tunnel: [w841] -> w57
    tunnel: [w840] -> w56
    tunnel: w53 -> [w839]
    tunnel: [w839] -> w54
    tunnel: w51 -> [w838]
    tunnel: [w838] -> w50
    tunnel: w48 -> [w837]
    tunnel: [w837] -> w47
    tunnel: w45 -> [w836]
    tunnel: [w836] -> w44
    tunnel: w42 -> [w835]
    tunnel: [w835] -> w41
    tunnel: w39 -> [w834]
    tunnel: [w834] -> w38
    tunnel: w36 -> [w833]
    tunnel: [w833] -> w35
    tunnel: w32 -> [w832]
    tunnel: [w832] -> w31
    tunnel: w27 -> [w831]
    tunnel: [w831] -> w26
    tunnel: w22 -> [w830]
    tunnel: [w830] -> w21
    tunnel: [w826] -> w9
    tunnel: [w825] -> w8
    tunnel: w7 -> [w824]
    tunnel: w4 -> [w823]
    tunnel: w98 -> [w895]
    tunnel: w97 -> [w894]
    tunnel: w94 -> [w893]
    tunnel: w93 -> [w892]
    tunnel: w91 -> [w891]
    tunnel: w88 -> [w890]
    tunnel: w82 -> [w889]
    tunnel: w81 -> [w888]
    tunnel: w78 -> [w887]
    tunnel: w77 -> [w886]
    tunnel: w73 -> [w885]
    tunnel: [w885] -> w72
    tunnel: [w884] -> w69
    tunnel: w68 -> [w884]
    tunnel: w67 -> [w883]
    tunnel: [w883] -> w65
    tunnel: w63 -> [w882]
    tunnel: [w882] -> w62
    tunnel: w60 -> [w881]
    tunnel: [w881] -> w59
    tunnel: [w880] -> w58
    tunnel: w57 -> [w880]
    tunnel: w56 -> [w879]
    tunnel: [w879] -> w55
    tunnel: w54 -> [w878]
    tunnel: [w878] -> w52
    tunnel: w50 -> [w877]
    tunnel: [w877] -> w49
    tunnel: [w876] -> w46
    tunnel: w47 -> [w876]
    tunnel: w44 -> [w875]
    tunnel: [w875] -> w43
    tunnel: w41 -> [w874]
    tunnel: [w874] -> w40
    tunnel: w38 -> [w873]
    tunnel: [w873] -> w37
    tunnel: w35 -> [w872]
    tunnel: [w872] -> w34
    tunnel: w31 -> [w871]
    tunnel: [w871] -> w29
    tunnel: w26 -> [w870]
    tunnel: [w870] -> w24
    tunnel: [w869] -> w23
    tunnel: w21 -> [w869]
    tunnel: w9 -> [w868]
    tunnel: w8 -> [w867]
    frame #0 {
      n215 = call-poly <vilib>:"DAQmx Write.vi"("task/channels in"=w824, "data"=FALSE, "error in"=w823) -> ("task out"=w828:refnum<k21>, "error out"=w829:errorcluster)  [unwired: 10 in, 1 out]
      n216 = call <vilib>:"DAQmx Stop Task.vi"("task/channels in"=w866, "error in"=w865) -> ("task out"=w864:refnum<k21>, "error out"=w863:errorcluster)  [unwired: 12 in]
      n217 = call <vilib>:"DAQmx Stop Task.vi"("task/channels in"=w862, "error in"=w861) -> ("task out"=w860:refnum<k21>, "error out"=w859:errorcluster)  [unwired: 12 in]
      n218 = call <vilib>:"DAQmx Stop Task.vi"("task/channels in"=w854, "error in"=w853) -> ("task out"=w852:refnum<k21>, "error out"=w851:errorcluster)  [unwired: 12 in]
      n219 = call <vilib>:"IMAQdx Close Camera.vi"("error in"=w845, "Session In"=w846) -> ()  [unwired: 9 in, 1 out]
      n220 = call "IMAQ AVI2 Close"("error in (no error)"=w849, "AVI Refnum"=w848) -> ("error out"=w847:errorcluster)  [unwired: 9 in]
      n221 = call <vilib>:"IMAQdx Close Camera.vi"("error in"=w849, "Session In"=w850) -> ()  [unwired: 9 in, 1 out]
      n222 = call <vilib>:"DAQmx Stop Task.vi"("task/channels in"=w857, "error in"=w840) -> ("task out"=w856:refnum<k21>, "error out"=w855:errorcluster)  [unwired: 12 in]
      n223 = call <vilib>:"DAQmx Stop Task.vi"("task/channels in"=w828, "error in"=w829) -> ("task out"=w826:refnum<k21>, "error out"=w825:errorcluster)  [unwired: 12 in]
    }
    frame #1 {
      n224 = call <vilib>:"DAQmx Clear Task.vi"("task in"=w868, "error in"=w867) -> ()  [unwired: 13 in, 1 out]
      n225 = call <vilib>:"DAQmx Clear Task.vi"("task in"=w895, "error in"=w894) -> ()  [unwired: 13 in, 1 out]
      n226 = call <vilib>:"DAQmx Clear Task.vi"("task in"=w893, "error in"=w892) -> ()  [unwired: 13 in, 1 out]
      n227 = call <vilib>:"IMAQdx Close Camera.vi"("error in"=w890, "Session In"=w891) -> ()  [unwired: 9 in, 1 out]
      n228 = call <vilib>:"DAQmx Clear Task.vi"("task in"=w887, "error in"=w886) -> ()  [unwired: 13 in, 1 out]
      n229 = call <vilib>:"DAQmx Clear Task.vi"("task in"=w889, "error in"=w888) -> ()  [unwired: 13 in, 1 out]
    }
  }
  n230 = call <vilib>:"IMAQ Extract Buffer.vi"("error in (no error)"=w34, "Buffer to extract"=-1, "IMAQ Session In"=w37) -> ("error out"=w473:errorcluster, "IMAQ Session Out"=w472:refnum<k11>)  [unwired: 7 out]
  n231 = Close File(refnum=w62, error in=w55) -> (path=w372:path)  [unwired: 1 out]
  n232 = Delete From Array(array=w46, length=1, index=0) -> (array with subset deleted=w277:u32[])  [unwired: 1 out]
  n233 = Delete From Array(array=w49, length=1, index=0) -> (array with subset deleted=w278:u32[])  [unwired: 1 out]
  n234 = Delete From Array(array=w43, length=1, index=0) -> (array with subset deleted=w203:u32[])  [unwired: 1 out]
  n235 = Delete From Array(array=w40, length=1, index=0) -> (array with subset deleted=w202:u32[])  [unwired: 1 out]
  n236 = Close File(refnum=w65, error in=w69) -> (path=w371:path, error out=w370:errorcluster)
  n237 = Close File(refnum=w59, error in=w58) -> (path=w199:path, error out=w198:errorcluster)
  n238 = Build Array(w277, w278) -> (w280:u32[][])
  n239 = call <vilib>:"IMAQ Close.vi"("error in (no error)"=w473, "IMAQ Session In"=w472) -> ("error out"=w474:errorcluster)  [unwired: 9 out]
  n240 = Build Array(w202, w203) -> (w205:u32[][])
  n241 = Array To Spreadsheet String(delimiter (Tab)=",", array=w278, 3:"%d" ("format string")) -> (spreadsheet string=w295:string)
  n242 = Transpose 2D Array(2D array=w280) -> (transposed array=w279:u32[][])
  n243 = Array To Spreadsheet String(delimiter (Tab)=",", array=w277, 3:"%d" ("format string")) -> (spreadsheet string=w296:string)
  n244 = Move(source path=w199, error in=w198, 10:"Target Path") -> (error out=w200:errorcluster)  [unwired: 2 in, 2 out]
  n245 = Move(source path=w371, error in=w370, 10:"Target Path") -> (error out=w368:errorcluster)  [unwired: 2 in, 2 out]
  n246 = Array To Spreadsheet String(delimiter (Tab)=",", array=w203, 3:"%d" ("format string")) -> (spreadsheet string=w206:string)
  n247 = Transpose 2D Array(2D array=w205) -> (transposed array=w204:u32[][])
  n248 = Move(source path=w23, error in=w72, 10:"Target Path") -> (error out=w367:errorcluster)  [unwired: 2 in, 2 out]
  n249 = Array To Spreadsheet String(delimiter (Tab)=",", array=w202, 3:"%d" ("format string")) -> (spreadsheet string=w207:string)
  n250 = for {
    N: w24 -> [_]
    tunnel: w29 -> [w899] mode=indexing
    shift-right: [w897] -> w374
    shift-left: w474 -> [w898]
    n251 = call "IMAQ Dispose"("All Images? (No)"=FALSE, "Image"=w899, "error in (no error)"=w898) -> ("error out"=w897:errorcluster)  [unwired: 3 out]
  }
  n252 = call <vilib>:"Trim Whitespace.vi"("string"=w296) -> ("trimmed string"=w192:string)  [unwired: 1 in]
  n253 = call <vilib>:"Trim Whitespace.vi"("string"=w295) -> ("trimmed string"=w191:string)  [unwired: 1 in]
  n254 = Number To Decimal String(number=w279) -> ()  [unwired: 1 in, 1 out]
  n255 = call <vilib>:"Trim Whitespace.vi"("string"=w207) -> ("trimmed string"=w193:string)  [unwired: 1 in]
  n256 = call <vilib>:"Trim Whitespace.vi"("string"=w206) -> ("trimmed string"=w194:string)  [unwired: 1 in]
  n257 = Number To Decimal String(number=w204) -> ()  [unwired: 1 in, 1 out]
  n258 = call <vilib>:"Simple Error Handler.vi"("error in (no error)"=w200) -> ()  [unwired: 1 in, 8 out]
  n259 = call <vilib>:"Simple Error Handler.vi"("error in (no error)"=w368) -> ()  [unwired: 1 in, 8 out]
  n260 = call <vilib>:"Simple Error Handler.vi"("error in (no error)"=w367) -> ()  [unwired: 1 in, 8 out]
  n261 = Build Array(w193, w194, w192, w191) -> (w190:string[])
  n262 = Move(source path=w372, error in=w374, 10:"Target Path") -> (error out=w373:errorcluster)  [unwired: 2 in, 2 out]
  n263 = TDMS Set Properties(5:w190, 7:string[] ["PupilCam_DroppedFrameIndex", "PupilCam_NumberDropped", "WhiskCam_DroppedFrameIndex", "WhiskCam_NumberDropped"] ("channel name(s) in (Untitled)"), 8:w55, 11:w52) -> (0:w302:errorcluster, 3:w301:refnum<k34>)  [unwired: 2 in, 2 out]
  n264 = TDMS Close(8:w302, 11:w301) -> (0:w375:errorcluster, 3:w364:path)
  n265 = Path To String(path=w364) -> (string=w366:string)
  n266 = call <vilib>:"Simple Error Handler.vi"("error in (no error)"=w373) -> ()  [unwired: 1 in, 8 out]
  n267 = TDMS Defragment(4:w375, 7:w364) -> (0:w361:errorcluster)
  n268 = Concatenate Strings(w366, "_index" ("string")) -> (w363:string)
  n269 = String To Path(string=w363) -> (path=w362:path)
  n270 = Move(source path=w364, error in=w361, 10:"Target Path") -> (error out=w369:errorcluster)  [unwired: 2 in, 2 out]
  n271 = Move(source path=w362, error in=w361, 10:"Target Path") -> (error out=w201:errorcluster)  [unwired: 2 in, 2 out]
  n272 = call <vilib>:"Simple Error Handler.vi"("error in (no error)"=w369) -> ()  [unwired: 1 in, 8 out]
  n273 = call <vilib>:"Simple Error Handler.vi"("error in (no error)"=w201) -> ()  [unwired: 1 in, 8 out]
